vi "Druckkorrektur.vi"(5 "output range":cluster{"output high":sgl, "output low":sgl}={"output high"=100.0, "output low"=-100.0} {"output low" format="%.2f"; "output high" format="%.2f"}, 6 "Output":sgl, 7 "Sollwert":sgl, 8 "Regler EIN":bool=TRUE, 9 "Auto?":bool, 10 "PID-Parameter":T1 {"Regler Toleranz -" format="%_2f"; "Regler Toleranz +" format="%_2f"; "D-Anteil" format="%_2f"; "I-Anteil" format="%_2f"; "P-Anteil" format="%_2f"}, 11 "Istwert":sgl) -> (3 "Interne Werte speichern":bool, 4 "Output":sgl)   [LabVIEW 2020, in "Regler.lvlib" / "Druckregler.lvlib"]
uses:
  Druckregler.lvlib
  Allgemein/Allgemein.lvlib
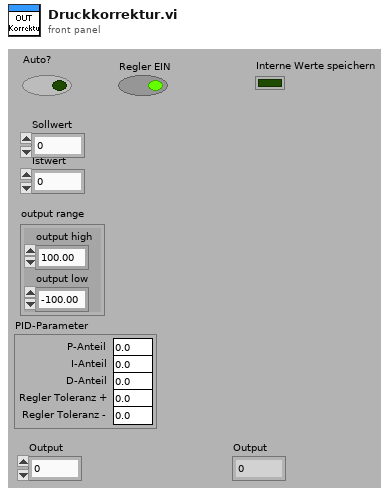
[diagram p1: front panel]
types:
  T1 = cluster{"P-Anteil":sgl, "I-Anteil":sgl, "D-Anteil":sgl, "Regler Toleranz +":sgl, "Regler Toleranz -":sgl}
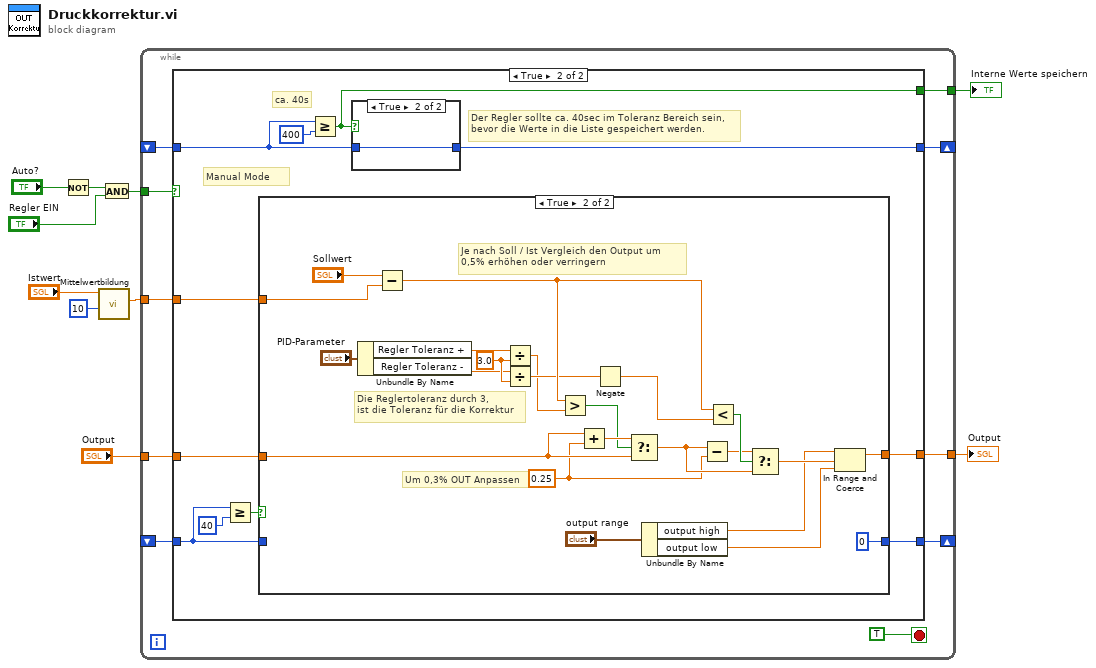
[diagram p0: block diagram]
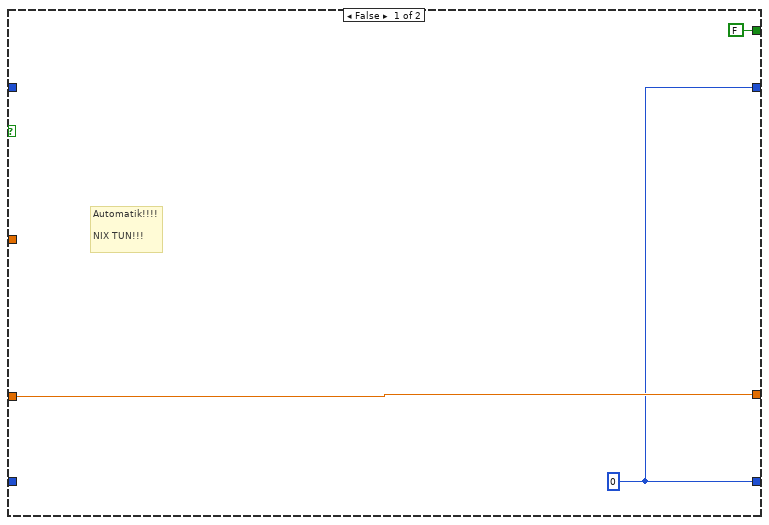
[diagram p2: hidden frame]
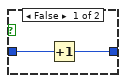
[diagram p3: hidden frame]
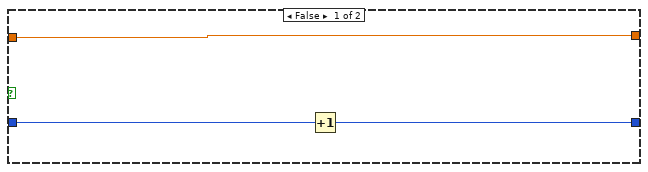
[diagram p4: hidden frame]
diagram:
  n1 = Not(x="Auto?") -> (.not. x?=w4:bool)
  n2 = call "Mittelwertbildung.vi"("Anzahl Werte"=u8 10, "Neuer Wert"="Istwert") -> ("gemittelter Wert"=w6:sgl)  [unwired: 7 in, 2 out]
  n3 = And(x=w4, y="Regler EIN") -> (x .and. y?=w3:bool)
  n4 = while {
    tunnel: w3 -> [w14]
    tunnel: [w20] -> w10
    tunnel: "Output" -> [w19]
    tunnel: w6 -> [w18]
    shift-right: [w17] -> _
    shift-left: _ -> [w16]
    shift-right: [w13] -> _
    shift-left: _ -> [w12]
    tunnel: [w11] -> w1
    stop <- TRUE stop-if-true
    n5 = case shown="True" w14 {
      tunnel: [w23 w34] -> w20
      tunnel: w19 -> [w23 w33]
      tunnel: w18 -> [_ w32]
      tunnel: [w21 w31] -> w17
      tunnel: w16 -> [_ w30]
      tunnel: [w21 w27] -> w13
      tunnel: w12 -> [_ w25]
      tunnel: [FALSE w24] -> w11
      frame False {
        w21 = u16 0 ("Anzahl Werte")
        # "Automatik!!!!\n\nNIX TUN!!!"
      }
      frame True {
        # "Der Regler sollte ca. 40sec im Toleranz Bereich sein,\nbevor die Werte in die Liste gespeichert werden."
        # "ca. 40s"
        # "Manual Mode"
        n6 = Greater Or Equal?(x=w30, y=u8 40) -> (x >= y?=w29:bool)
        n7 = case shown="True" w29 {
          tunnel: [w40 w63] -> w34
          tunnel: w33 -> [w40 w52]
          tunnel: w32 -> [_ w62]
          tunnel: [w38 u16 0 ("Anzahl Werte")] -> w31
          tunnel: w30 -> [w39 _]
          frame False {
            n8 = Increment(x=w39) -> (x+1=w38:u16)
          }
          frame True {
            w48 = sgl 3.0 ("y")
            w50 = sgl 0.25 ("y")
            # "Die Reglertoleranz durch 3,\nist die Toleranz für die Korrektur"
            # "Um 0,3% OUT Anpassen"
            # "Je nach Soll / Ist Vergleich den Output um \n0,5% erhöhen oder verringern"
            n9 = Unbundle By Name("PID-Parameter") -> ("Regler Toleranz +"=w46:sgl, "Regler Toleranz -"=w47:sgl)
            n10 = Subtract(x="Sollwert", y=w62) -> (x-y=w57:sgl)
            n11 = Divide(x=w46, y=w48) -> (x/y=w44:sgl)
            n12 = Divide(x=w47, y=w48) -> (x/y=w49:sgl)
            n13 = Greater?(x=w57, y=w44) -> (0:w58:bool)
            n14 = Add(x=w52, y=w50) -> (x+y=w59:sgl)
            n15 = Negate(x=w49) -> (-x=w43:sgl)
            n16 = Select(t=w59, s=w58, f=w52) -> (s? t:f=w51:sgl)
            n17 = Unbundle By Name("output range") -> ("output high"=w42:sgl, "output low"=w41:sgl)
            n18 = Subtract(x=w51, y=w50) -> (x-y=w55:sgl)
            n19 = Less?(x=w57, y=w43) -> (x < y?=w56:bool)
            n20 = Select(t=w55, s=w56, f=w51) -> (s? t:f=w53:sgl)
            n21 = In Range and Coerce(upper limit=w42, x=w53, lower limit=w41) -> (coerced(x)=w63:sgl)  [unwired: 1 out]
          }
        }
        n22 = Greater Or Equal?(x=w25, y=u16 400) -> (x >= y?=w24:bool)
        n23 = case shown="True" w24 {
          tunnel: [w36 w37] -> w27
          tunnel: w25 -> [w35 w37]
          frame False {
            n24 = Increment(x=w35) -> (x+1=w36:u16)
          }
          frame True {
          }
        }
      }
    }
  }
  "Output" <- w10
  "Interne Werte speichern" <- w1
